vi "Dashboard Main.vi"() -> ()   [LabVIEW 2012]
uses:
  <vilib>/event_ctls.llb/eventvkey.ctl
  <vilib>/Utility/config.llb/Read Key (String).vi
  <vilib>/Utility/config.llb/Read Key (I32).vi
  <vilib>/Utility/config.llb/Write Key (String).vi
  <vilib>/Utility/config.llb/Write Key (I32).vi
  <vilib>/Utility/config.llb/NI_LVConfig.lvlib
panel:
  out "Mode":T1(ring)=enum."Auto Disabled"
  in  "Viewer":enum32{"Camera Image", "Variables"}(tab)
  out "Mbps":dbl format="%#.1g"
  in  "Enable":bool=TRUE
  in  "DB Camera Config":bool
  out "Mbps":bool
  out "fps":dbl format="%#.1g"
  out "Image Error Message":string="Timeout in Camera Communications"
  out "Camera Image":T2(plugin-control)
  out "Camera Image 2":T2(plugin-control)
  in  "Camera Settings":T3={"Frame Rate"=15, "Compression"=30, "Size"=1} {"Frame Rate" scale=1.0..30.0; "Size" items=["640x480", "320x240", "160x120"]}
  out "Camera IP 2":string
  out "Camera IP":string
  out "fps 2":dbl format="%#.1g"
  out "Mbps 2":dbl format="%#.1g"
  in  "Enable 2":bool=TRUE
  in  "FR":i32=15
  out "Tree":string(tree)
  in  "Dashboard Tab":enum32{"Operation", "Test", "Checklist"}(tab)
  in  "Auton Selector":T4(radio)
  in  "Auton Refresh":bool
  out "AutonFiles":string[](array[string])
  out "Refnum out":T2(plugin-control)
  in  "Score Limits":T5={"Rect Coverage"=60.0, "X Edge Strength"=40.0, "Y Edge Strength"=60.0, "Center"=75.0, "Outer"=75.0}
  in  "Range":cluster{"Lower value":sgl, "Upper value":sgl}={"Lower value"=150.0, "Upper value"=255.0}
  out "Out Circle Info":cluster{dbl, dbl}
  out "Out Target Info":cluster{"X":dbl, "Y":dbl, "Distance (ft)":dbl}
  in  "Slider":dbl(slide) scale=0.0..100.0 scale format="%#_3g"
  in  "On/Off":bool caption="Solenoid"
  in  "Test Name":u16(ring) items=["Select the test to run...", "Example Test", "-------------------------------", "List of tests is built in robot code.", "Replace with your own automated tests."]
  in  "Test Tree":string(tree)
  in  "Motor":cluster{"Value":dbl, "Enable":bool} {"Value" scale=-1.0..1.0 scale format="%#_3g"}
  out "Progress":T6 {"Test Progress" scale=0.0..100.0}
  in  "Rev/Fwd":cluster{"Forward":bool, "Reverse":bool}
  in  "Ring":u16(ring) items=["Auto", "Fixed indoor", "Fixed outdoor 1", "Fixed outdoor 2", "Fixed fluorescent 1", "Fixed fluorescent 2", "Hold current"]
  in  "Listbox":i32(listbox)
  out "Robot IP":string
  out "Battery Value":dbl(slide) scale=0.0..14.0 scale format="%#_2e"
  out "Battery":sgl(graph)
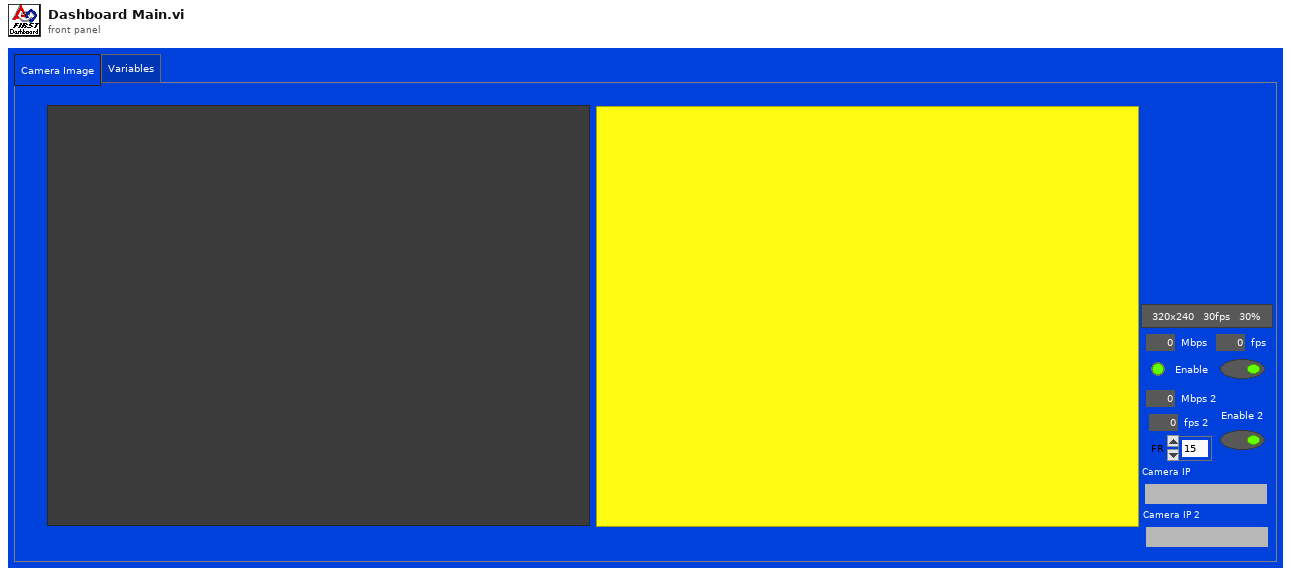
[diagram p1: front panel]
types:
  T1 = enum8{"Tele-Op Disabled", "Tele-Op Enabled", "Auto Disabled", "Auto Enabled", "Test Disabled", "Test Enabled", ""}
  T2 = typedef "IMAQ Image.ctl" = refnum<image>
  T3 = cluster{"Frame Rate":i32, "Compression":i32, "Size":u16}
  T4 = enum32{"Boolean 1", "Boolean 2", "Boolean 3", "Boolean 4", "Boolean 5", "Boolean 6", "Boolean 7", "Boolean 8", "Boolean 9", "Boolean 10"}
  T5 = cluster{"Rect Coverage":dbl, "X Edge Strength":dbl, "Y Edge Strength":dbl, "Center":dbl, "Outer":dbl}
  T6 = cluster{"Test Progress":u8, "Test Progress Text":string}
  T7 = typedef "Image Type" = u32
  T8 = cluster{"Competition mode":bool, "Robot Link":bool, "Autonomous":bool, "Enabled":bool, "E-Stop":bool, "Simulated":bool, "TestMode":bool, "Docked Window":bool}
  T9 = typedef "LVRectTypeDef.ctl" = cluster{"Left":i16, "Top":i16, "Right":i16, "Bottom":i16}
  T10 = typedef "NI_LVConfig.lvlib/Config Data RefNum.ctl" = refnum<k1>
  T11 = typedef "eventvkey.ctl" = enum16{"ASCII", "Enter", "Return", "Shift", "Ctrl", "Alt", "Cmd", "Opt", "Caps", "NumLock", "Clear", "Break", "Up", "Down", "Left", "Right", "Insert", "Delete", "Home", "End", "PageUp", "PageDown", "Escape", "Help", "Pause", "ScrollLock", "F1", "F2", "F3", "F4", "F5", "F6", "F7", "F8", "F9", "F10", "F11", "F12", "F13", "F14", "F15", "F16", "F17", "F18", "F19", "F20", "F21", "F22", "F23", "F24", "Play", "VolumeUp", "VolumeDown", "Mute", "Two Byte Char"}
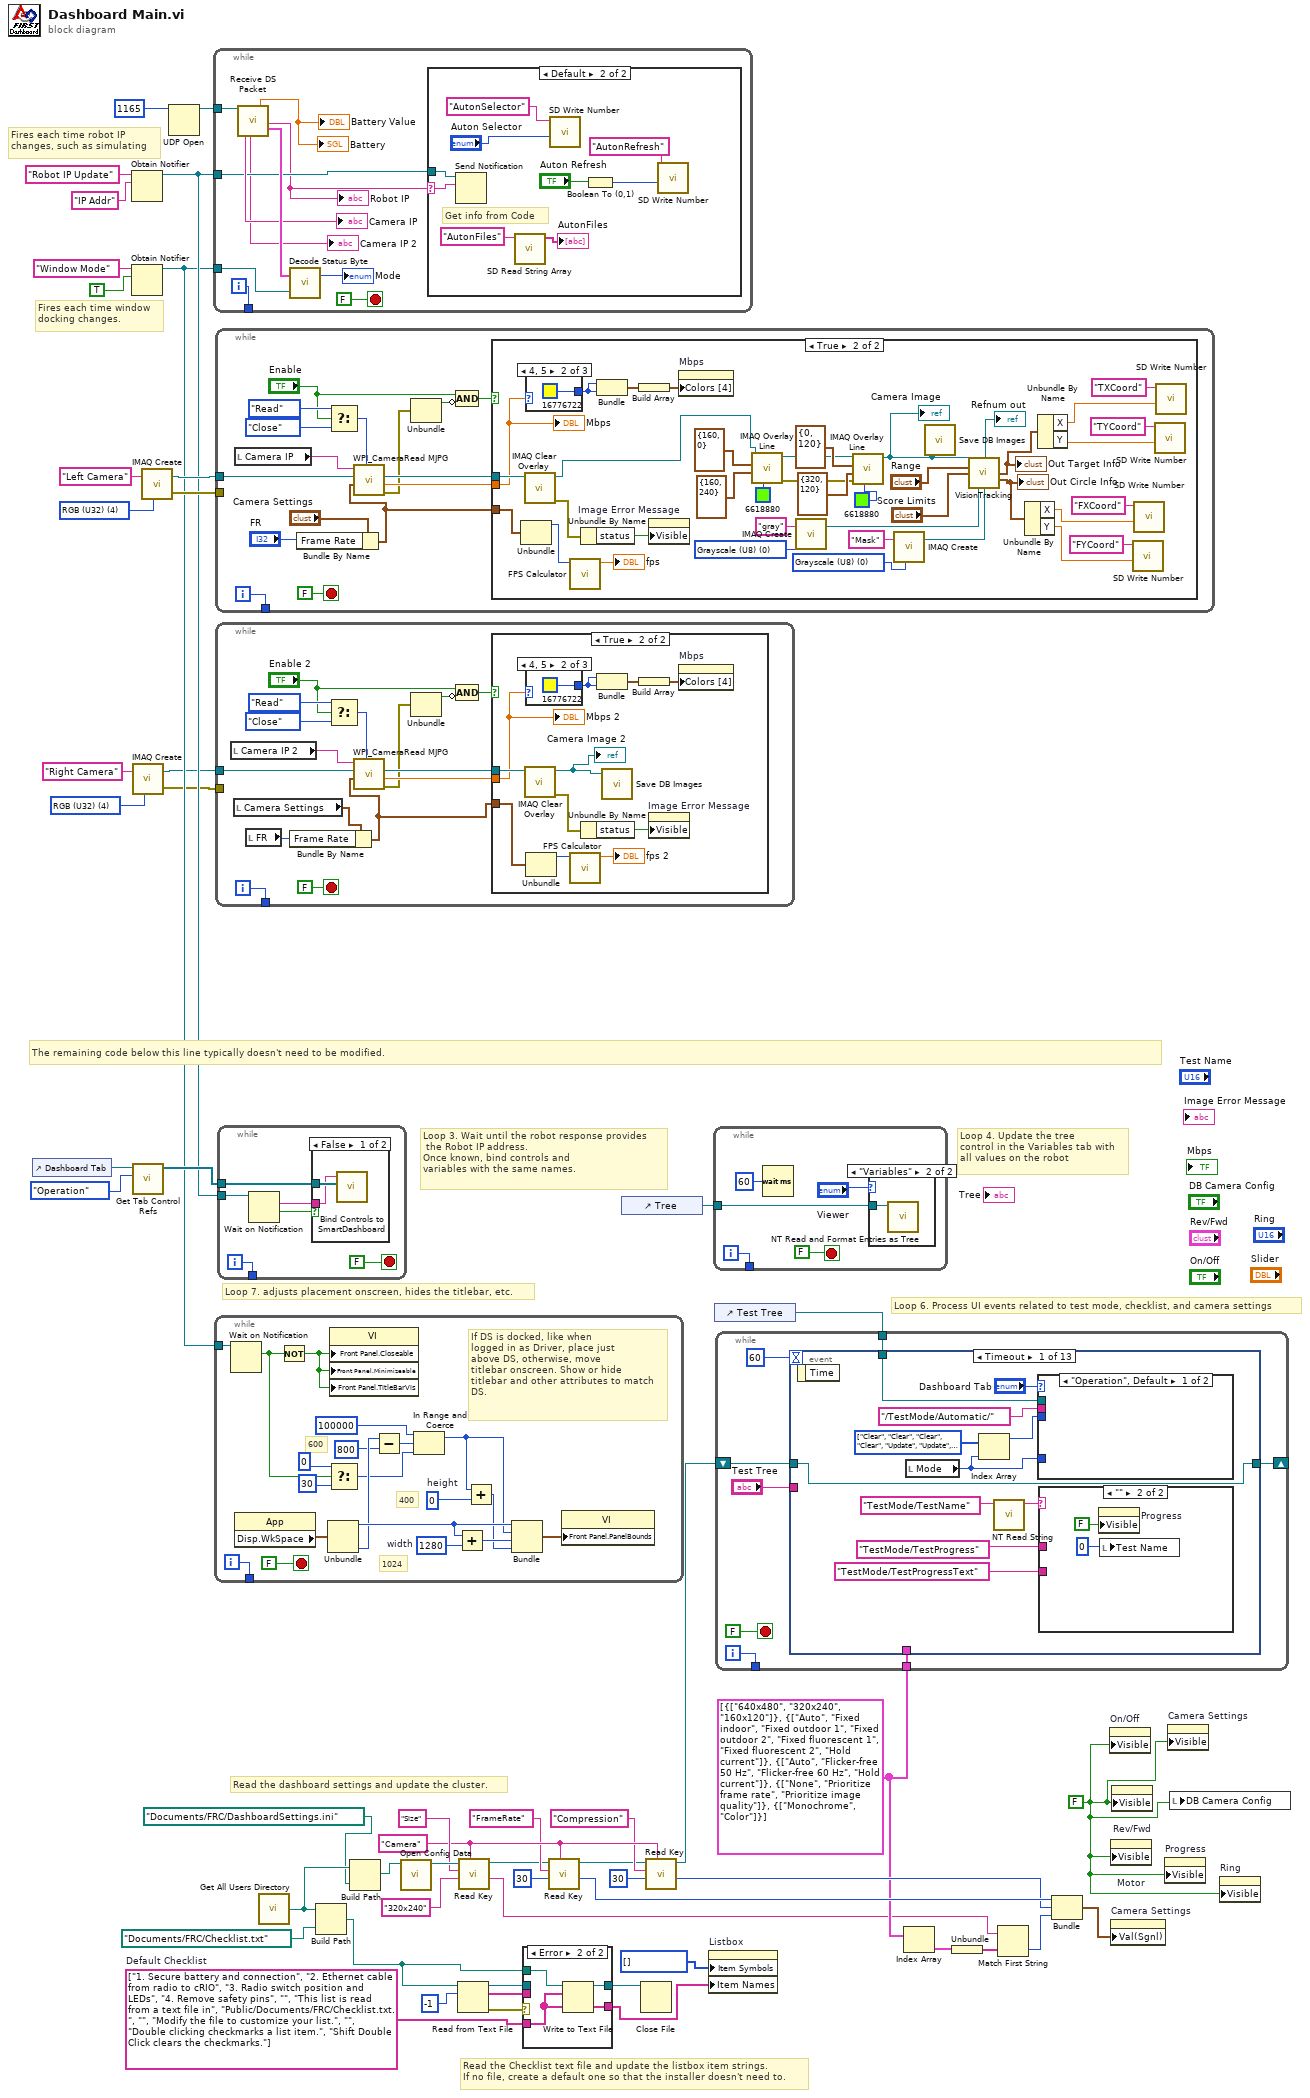
[diagram p0: block diagram]
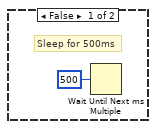
[diagram p2: hidden frame]
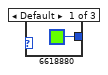
[diagram p3: hidden frame]
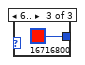
[diagram p4: hidden frame]
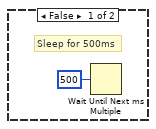
[diagram p6: hidden frame]
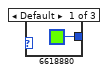
[diagram p7: hidden frame]
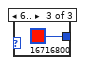
[diagram p8: hidden frame]
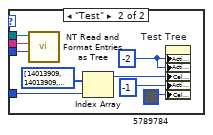
[diagram p10: hidden frame]
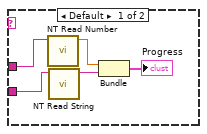
[diagram p11: hidden frame]
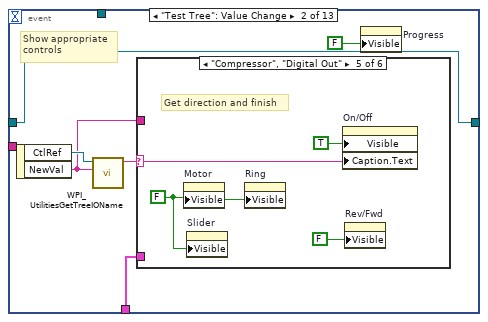
[diagram p12: hidden frame]
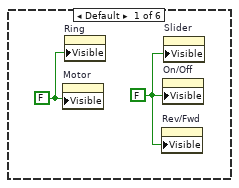
[diagram p13: hidden frame]
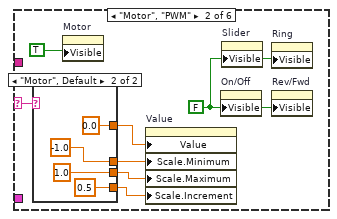
[diagram p14: hidden frame]
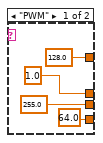
[diagram p15: hidden frame]
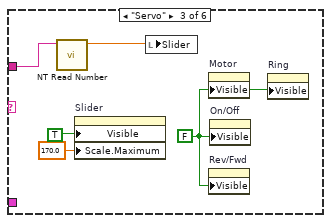
[diagram p16: hidden frame]
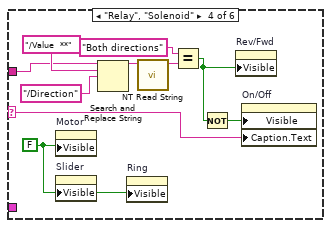
[diagram p17: hidden frame]
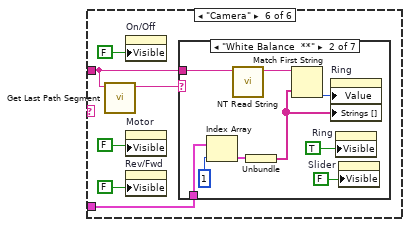
[diagram p18: hidden frame]
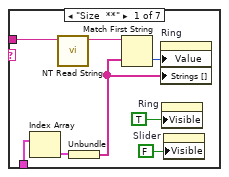
[diagram p19: hidden frame]
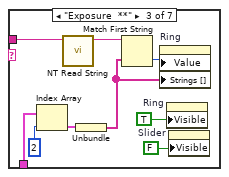
[diagram p20: hidden frame]
diagram:
  w3 = T7 4 items=["Grayscale (U8)", "Grayscale (I16)", "Grayscale (SGL)", "Complex (CSG)", "RGB (U32)", "HSL (U32)", "RGB (U64)"] ("Image Type")
  w25 = "Camera"
  w17 = cluster{string[]}[] [{["640x480", "320x240", "160x120"]}, {["Auto", "Fixed indoor", "Fixed outdoor 1", "Fixed outdoor 2", "Fixed fluorescent 1", "Fixed fluorescent 2", "Hold current"]}, {["Auto", "Flicker-free 50 Hz", "Flicker-free 60 Hz", "Hold current"]}, {["None", "Prioritize frame rate", "Prioritize image quality"]}, {["Monochrome", "Color"]}]
  w33 = string[] ["1. Secure battery and connection", "2. Ethernet cable from radio to cRIO", "3. Radio switch position and LEDs", "4. Remove safety pins", "", "This list is read from a text file in", "Public/Documents/FRC/Checklist.txt.", "", "Modify the file to customize your list.", "", "Double clicking checkmarks a list item.", "Shift Double Click clears the checkmarks."]  # Default Checklist
  w31 = FALSE ("Visible")
  w52 = T7 4 items=["Grayscale (U8)", "Grayscale (I16)", "Grayscale (SGL)", "Complex (CSG)", "RGB (U32)", "HSL (U32)", "RGB (U64)"] ("Image Type")
  # "Fires each time robot IP\nchanges, such as simulating"
  # "Fires each time window\ndocking changes."
  # "Read the Checklist text file and update the listbox item strings.\nIf no file, create a default one so that the installer doesn't need to."
  # "The remaining code below this line typically doesn't need to be modified."
  # "Loop 6. Process UI events related to test mode, checklist, and camera settings"
  # "Read the dashboard settings and update the cluster."
  # "Loop 4. Update the tree\ncontrol in the Variables tab with\nall values on the robot"
  # "Loop 3. Wait until the robot response provides\n the Robot IP address.\nOnce known, bind controls and\nvariables with the same names."
  # "Loop 7. adjusts placement onscreen, hides the titlebar, etc."
  n1 = control-ref of="Dashboard Tab"() -> (w47:refnum<vi>)
  n2 = Obtain Notifier(name (unnamed)="Robot IP Update", notification data type="IP Addr" ("name (unnamed)")) -> (notifier out=w44:refnum<notifier>)  [unwired: 2 in, 2 out]
  n3 = Obtain Notifier(name (unnamed)="Window Mode", notification data type=TRUE) -> (notifier out=w37:refnum<notifier>)  [unwired: 2 in, 2 out]
  n4 = call "IMAQ Create"("Image Name"="Right Camera", "Image Type"=w3) -> ("New Image"=w2:T2, "error out"=w1:errorcluster)  [unwired: 2 in, 1 out]
  n5 = call <vilib>:"Get Tab Control Refs.vi"("Page Index"=enum32{"Operation", "Test"}."Operation" ("Dashboard Tab"), "TabControl in"=w47) -> ("ControlsOnPage"=w48:refnum<vi>[])  [unwired: 9 in]
  n6 = call "IMAQ Create"("Image Name"="Left Camera", "Image Type"=w52) -> ("New Image"=w50:T2, "error out"=w49:errorcluster)  [unwired: 2 in, 1 out]
  n7 = UDP Open(11:u16 1165 ("port")) -> (port=w53:refnum<k16>)  [unwired: 2 in, 4 out]
  n8 = while {
    tunnel: w53 -> [w63]
    tunnel: w44 -> [w57]
    tunnel: w37 -> [w61]
    tunnel: [w58] -> _
    i -> [w58]
    stop <- FALSE stop-if-true
    n9 = call "Receive DS Packet.vi"("Recv Socket"=w63) -> ("Camera IP Address"=→"Camera IP":string, "Camera IP Address 2"=→"Camera IP 2":string, "Battery"=→"Battery" →"Battery Value":sgl, "Robot IP Address"=w56:string, "Status"=w64:T8)  [unwired: 8 in, 6 out]
    "Robot IP" <- w56
    n10 = call "Decode Status Byte.vi"("Window Mode Notifier"=w61, "Status"=w64) -> ("Mode"=→"Mode":T1)  [unwired: 1 out]
    n11 = case shown="Default" w56 {
      selector: w56 -> [_ w73]
      tunnel: w57 -> [_ w74]
      frame "0.0.0.0" {
        # "Robot not responding, don't poll the variables"
      }
      frame Default {
        # "Get info from Code"
        n12 = Send Notification(notification=w73, notifier=w74) -> ()  [unwired: 1 in, 2 out]
        n13 = call <vilib>:"SD Read String Array.vi"("Name"="AutonFiles") -> ("String Array"=→"AutonFiles":string[])  [unwired: 9 in, 1 out]
        n14 = call <vilib>:"SD Write Number.vi"("Numeric"="Auton Selector", "Name"="AutonSelector") -> ()  [unwired: 8 in, 2 out]
        n15 = Boolean To (0,1)(Boolean="Auton Refresh") -> (0, 1=w67:i16)
        n16 = call <vilib>:"SD Write Number.vi"("Numeric"=w67, "Name"="AutonRefresh") -> ()  [unwired: 8 in, 2 out]
      }
    }
  }
  n17 = while {
    tunnel: w37 -> [w93]
    tunnel: [w91] -> _
    i -> [w91]
    stop <- FALSE stop-if-true
    w83 = 1280  # width
    w86 = 0  # height
    # "600"
    # "1024"
    # "400"
    # "If DS is docked, like when\nlogged in as Driver, place just\nabove DS, otherwise, move\ntitlebar onscreen. Show or hide\ntitlebar and other attributes to match\nDS."
    n18 = Wait on Notification(notifier=w93) -> (notification=w78:bool)  [unwired: 3 in, 3 out]
    n19 = property class="App"() -> ("Disp.WkSpace"=w89:T9)  [unwired: 2 in, 2 out]
    n20 = Not(x=w78) -> (.not. x?=w92:bool)
    n21 = Unbundle(w89) -> ("Left"=w87:i16, "Bottom"=w84:i16)  [unwired: 2 out]
    n22 = Select(t=0, s=w78, f=30) -> (s? t:f=w77:i32)
    n23 = property class="VI"("Front Panel.Closeable"=w92, "Front Panel.Minimizeable"=w92, "Front Panel.TitleBarVis"=w92) -> ()  [unwired: 2 in, 2 out]
    n24 = Subtract(x=w84, y=800) -> (x-y=w81:i32)
    n25 = In Range and Coerce(upper limit=100000, x=w81, lower limit=w77) -> (coerced(x)=w75:i32)  [unwired: 1 out]
    n26 = Add(x=w87, y=w83) -> (x+y=w88:i32)
    n27 = Add(x=w75, y=w86) -> (x+y=w85:i32)
    n28 = Bundle("Left"=w87, w75, w88, w85) -> (w90:cluster{"Left":i16, i32, i32, i32})  [unwired: 1 out]
    n29 = property class="VI"("Front Panel.PanelBounds"=w90) -> ()  [unwired: 2 in, 2 out]
  }
  n30 = while {
    tunnel: w50 -> [w107]
    tunnel: w49 -> [_]
    tunnel: [w109] -> _
    i -> [w109]
    stop <- FALSE stop-if-true
    n31 = local read "Camera IP"() -> (w108:string)
    n32 = Bundle By Name(cluster="Camera Settings", "Frame Rate"="FR") -> (w95:T3)
    n33 = Select(t=enum16{"Read", "Reopen", "Close"}."Read" ("Operation"), s="Enable", f=enum16{"Read", "Reopen", "Close"}."Close" ("Operation")) -> (s? t:f=w102:enum16{"Read", "Reopen", "Close"})
    n34 = call <vilib>:"WPI_CameraRead MJPG.vi"("Operation"=w102, "Camera Settings"=w95, "Image"=w107, "address"=w108) -> ("error out"=w101:errorcluster, "Bandwidth (kbps)"=w105:dbl, "Image Out"=w106:T2)  [unwired: 5 in]
    n35 = Unbundle(w101) -> ("status"=w99:bool)  [unwired: 2 out]
    n36 = Compound Arithmetic op=AND("Enable", invert w99) -> (w98:bool)
    n37 = case shown="True" w98 {
      tunnel: w95 -> [_ w142]
      tunnel: w106 -> [_ w145]
      tunnel: w105 -> [_ w144]
      frame False {
        # "Sleep for 500ms"
        n38 = Wait Until Next ms Multiple(millisecond multiple=u32 500) -> ()  [unwired: 1 out]
      }
      frame True {
        w126 = T7 0 items=["Grayscale (U8)", "Grayscale (I16)", "Grayscale (SGL)", "Complex (CSG)", "RGB (U32)", "HSL (U32)", "RGB (U64)", "Grayscale (U16)"] ("Image Type")
        w128 = T7 0 items=["Grayscale (U8)", "Grayscale (I16)", "Grayscale (SGL)", "Complex (CSG)", "RGB (U32)", "HSL (U32)", "RGB (U64)", "Grayscale (U16)"] ("Image Type")
        n39 = Unbundle(w142) -> ("Frame Rate"=w133:i32)  [unwired: 2 out]
        n40 = call "IMAQ Clear Overlay"("Image"=w145) -> ("error out"=w149:errorcluster, "Image Out"=w134:T2)  [unwired: 2 in, 7 out]
        n41 = case shown="4, 5" w144 {
          tunnel: [u32 6618880 ("Color Box") u32 16776722 ("Color Box") u32 16716800 ("Color Box")] -> w146
          frame Default {
          }
          frame 4, 5 {
          }
          frame 6.. {
          }
        }
        n42 = call "FPS Calculator.vi"("Average Count"=w133) -> ("fps"=→"fps":dbl)  [unwired: 10 in]
        n43 = Unbundle By Name(w149) -> ("status"=w150:bool)
        n44 = Bundle("Color Box"=w146, "Color Box"=w146) -> (w148:cluster{"Color Box":u32, "Color Box":u32})  [unwired: 1 out]
        n45 = Build Array(w148) -> (w147:cluster{"Color Box":u32, "Color Box":u32}[])
        n46 = property on="Image Error Message" class="Str"("Visible"=w150) -> ()  [unwired: 2 in, 2 out]
        n47 = property on="Mbps" class="Bool (strict)"("Colors [4]"=w147) -> ()  [unwired: 2 in, 2 out]
        n48 = call "IMAQ Overlay Line"("Color"=u32 6618880, "End Point"=cluster{"X":i32, "Y":i32} {"X"=160, "Y"=240}, "Start Point"=cluster{"X":i32, "Y":i32} {"X"=160, "Y"=0}, "Image"=w134) -> ("error out"=w139:errorcluster, "Image Out"=w138:T2)  [unwired: 6 in]
        n49 = call "IMAQ Create"("Image Name"="gray", "Image Type"=w128) -> ("New Image"=w124:T2)  [unwired: 3 in, 1 out]
        n50 = call "IMAQ Overlay Line"("Color"=u32 6618880, "error in (no error)"=w139, "End Point"=cluster{"X":i32, "Y":i32} {"X"=320, "Y"=120}, "Start Point"=cluster{"X":i32, "Y":i32} {"X"=0, "Y"=120}, "Image"=w138) -> ("Image Out"=w131:T2)  [unwired: 5 in, 1 out]
        "Camera Image" <- w131
        n51 = call "IMAQ Create"("Image Name"="Mask", "Image Type"=w126) -> ("New Image"=w125:T2)  [unwired: 3 in, 1 out]
        n52 = call "Save DB Images.vi"("Image"=w131) -> ()  [unwired: 2 in, 1 out]
        n53 = call "VisionTracking.vi"("Refnum in"=w131, "Range"="Range", "Score Limits"="Score Limits", "New Image 2"=w124, "New Image"=w125) -> ("Refnum out"=→"Refnum out":T2, "Out Target Info"=w121:cluster{"X":dbl, "Y":dbl, "Distance (ft)":dbl}, "Out Cirlcle Info"=w114:cluster{"X":dbl, "Y":dbl})  [unwired: 8 in]
        "Out Target Info" <- w121
        "Out Circle Info" <- w114
        n54 = Unbundle By Name(w114) -> ("X"=w113:dbl, "Y"=w112:dbl)
        n55 = Unbundle By Name(w121) -> ("X"=w118:dbl, "Y"=w117:dbl)
        n56 = call <vilib>:"SD Write Number.vi"("Numeric"=w112, "Name"="FYCoord") -> ()  [unwired: 8 in, 2 out]
        n57 = call <vilib>:"SD Write Number.vi"("Numeric"=w113, "Name"="FXCoord") -> ()  [unwired: 8 in, 2 out]
        n58 = call <vilib>:"SD Write Number.vi"("Numeric"=w117, "Name"="TYCoord") -> ()  [unwired: 8 in, 2 out]
        n59 = call <vilib>:"SD Write Number.vi"("Numeric"=w118, "Name"="TXCoord") -> ()  [unwired: 8 in, 2 out]
        "Mbps" <- w144
      }
    }
  }
  n60 = while {
    tunnel: w2 -> [w166]
    tunnel: [w168] -> _
    tunnel: w1 -> [_]
    i -> [w168]
    stop <- FALSE stop-if-true
    n61 = local read "Camera IP 2"() -> (w167:string)
    n62 = local read "Camera Settings"() -> (w155:T3)
    n63 = local read "FR"() -> (w156:i32)
    n64 = Bundle By Name(cluster=w155, "Frame Rate"=w156) -> (w154:T3)
    n65 = Select(t=enum16{"Read", "Reopen", "Close"}."Read" ("Operation"), s="Enable 2", f=enum16{"Read", "Reopen", "Close"}."Close" ("Operation")) -> (s? t:f=w161:enum16{"Read", "Reopen", "Close"})
    n66 = call <vilib>:"WPI_CameraRead MJPG.vi"("Operation"=w161, "Camera Settings"=w154, "Image"=w166, "address"=w167) -> ("error out"=w160:errorcluster, "Bandwidth (kbps)"=w164:dbl, "Image Out"=w165:T2)  [unwired: 5 in]
    n67 = Unbundle(w160) -> ("status"=w158:bool)  [unwired: 2 out]
    n68 = Compound Arithmetic op=AND("Enable 2", invert w158) -> (w157:bool)
    n69 = case shown="True" w157 {
      tunnel: w154 -> [_ w173]
      tunnel: w165 -> [_ w176]
      tunnel: w164 -> [_ w175]
      frame False {
        # "Sleep for 500ms"
        n70 = Wait Until Next ms Multiple(millisecond multiple=u32 500) -> ()  [unwired: 1 out]
      }
      frame True {
        n71 = call "IMAQ Clear Overlay"("Image"=w176) -> ("error out"=w180:errorcluster, "Image Out"=w171:T2)  [unwired: 2 in, 7 out]
        "Camera Image 2" <- w171
        n72 = case shown="4, 5" w175 {
          tunnel: [u32 6618880 ("Color Box") u32 16776722 ("Color Box") u32 16716800 ("Color Box")] -> w177
          frame Default {
          }
          frame 4, 5 {
          }
          frame 6.. {
          }
        }
        n73 = Unbundle(w173) -> ("Frame Rate"=w172:i32)  [unwired: 2 out]
        n74 = call "FPS Calculator.vi"("Average Count"=w172) -> ("fps"=→"fps 2":dbl)  [unwired: 10 in]
        n75 = Unbundle By Name(w180) -> ("status"=w181:bool)
        n76 = Bundle("Color Box"=w177, "Color Box"=w177) -> (w179:cluster{"Color Box":u32, "Color Box":u32})  [unwired: 1 out]
        n77 = call "Save DB Images.vi"("Image"=w171) -> ()  [unwired: 2 in, 1 out]
        n78 = Build Array(w179) -> (w178:cluster{"Color Box":u32, "Color Box":u32}[])
        n79 = property on="Image Error Message" class="Str"("Visible"=w181) -> ()  [unwired: 2 in, 2 out]
        n80 = property on="Mbps" class="Bool (strict)"("Colors [4]"=w178) -> ()  [unwired: 2 in, 2 out]
        "Mbps 2" <- w175
      }
    }
  }
  n81 = while {
    tunnel: w48 -> [w190]
    tunnel: w44 -> [w187]
    tunnel: [w185] -> _
    i -> [w185]
    stop <- FALSE stop-if-true
    n82 = Wait on Notification(notifier=w187) -> (notification=w186:string, timed out?=w188:bool)  [unwired: 3 in, 2 out]
    n83 = case shown="False" w188 {
      tunnel: w190 -> [w192 _]
      tunnel: w186 -> [w191 _]
      frame False {
        n84 = call <vilib>:"Bind Controls to SmartDashboard.vi"("Bound Control Refs"=w192, "Server IP Address"=w191) -> ()  [unwired: 10 in]
      }
      frame True {
      }
    }
  }
  n85 = call "Get All Users Directory.vi"() -> ("All User Path"=w30:path)
  n86 = Build Path(base path=w30, name or relative path=path "Documents/FRC/Checklist.txt") -> (appended path=w34:path)
  n87 = Build Path(base path=w30, name or relative path=path "Documents/FRC/DashboardSettings.ini") -> (appended path=w29:path)
  n88 = call <vilib>:"Open Config Data.vi"("configuration file path"=w29) -> ("refnum"=w28:T10)  [unwired: 8 in, 2 out]
  n89 = Read from Text File(file (use dialog)=w34, count=-1 ("timeout ms (25000)")) -> (refnum out=w12:refnum<file>, text=w35:string[], error out=w36:errorcluster)  [unwired: 2 in, 1 out]
  n90 = call-poly <vilib>:"Read Key.vi"("section"=w25, "default value"="320x240", "key"="Size", "refnum"=w28) -> ("value"=w15:string, "refnum out"=w10:T10)  [unwired: 2 in, 4 out]
  n91 = case shown="Error" w36 {
    tunnel: w35 -> [w194 _]
    tunnel: [w194 w196] -> w32
    tunnel: w33 -> [_ w196]
    tunnel: w34 -> [_ w197]
    tunnel: [w193 w195] -> w11
    tunnel: w12 -> [w193 _]
    frame No Error {
    }
    frame Error {
      n92 = Write to Text File(file (use dialog)=w197, text=w196) -> (refnum out=w195:refnum<file>)  [unwired: 2 in, 2 out]
    }
  }
  n93 = call-poly <vilib>:"Read Key.vi"("section"=w25, "default value"=30, "key"="FrameRate", "refnum"=w10) -> ("value"=w20:i32, "refnum out"=w9:T10)  [unwired: 1 in, 5 out]
  n94 = control-ref of="Tree"() -> (w6:refnum<vi>)
  n95 = Close File(refnum=w11) -> ()  [unwired: 1 in, 2 out]
  n96 = call-poly <vilib>:"Read Key.vi"("section"=w25, "default value"=30, "key"="Compression", "refnum"=w9) -> ("value"=w19:i32, "refnum out"=w7:T10)  [unwired: 1 in, 5 out]
  n97 = property on="Listbox" class="LstBox (strict)"("Item Symbols"=i32[] [], "Item Names"=w32) -> ()  [unwired: 2 in, 2 out]
  n98 = while {
    tunnel: [w199] -> _
    tunnel: w6 -> [w198]
    i -> [w199]
    stop <- FALSE stop-if-true
    n99 = Wait (ms)(milliseconds to wait=u32 60) -> ()  [unwired: 1 out]
    n100 = case shown="\"Variables\"" "Viewer" {
      tunnel: w198 -> [_ w203]
      frame Default {
      }
      frame "Variables" {
        n101 = call <vilib>:"NT Read and Format Entries as Tree.vi"("Tree Refnum"=w203) -> ()  [unwired: 9 in, 2 out]
      }
    }
  }
  n102 = control-ref of="Test Tree"() -> (w5:refnum<vi>)
  n103 = while {
    tunnel: w17 -> [w208]
    shift-right: [w207] -> _
    shift-left: w7 -> [w206]
    tunnel: [w205] -> _
    tunnel: w5 -> [w204]
    i -> [w205]
    stop <- FALSE stop-if-true
    n104 = event shown="[0] Timeout" {
      selector: _ -> [_ _ _ _ _ _ _ _ _ _ _ _ _]
      dyn-events: _ -> [_ _ _ _ _ _ _ _ _ _ _ _ _]
      timeout: u32 60 ("milliseconds to wait") -> [_ _ _ _ _ _ _ _ _ _ _ _ _]
      tunnel: w204 -> [w218 _ _ _ _ _ _ _ _ _ _ _ _]
      tunnel: "Test Tree" -> [_ _ _ _ _ _ _ _ w412 w420 w422 w426 w434]
      tunnel: w208 -> [_ w240 _ _ _ _ w376 w406 _ _ _ _ _]
      tunnel: [w212 w239 _ w342 w350 w362 w375 w399 w411 w418 w421 w425 w433] -> w207
      tunnel: w206 -> [w212 w239 _ w342 w350 w362 w374 w399 w411 w418 w421 w425 w433]
      event Timeout {
        w217 = enum16{"Update", "Clear"}[] [enum."Clear", enum."Clear", enum."Clear", enum."Clear", enum."Update", enum."Update", enum."Clear"] items=["Update", "Clear"]
        n105 = event-data() -> ()  [unwired: 1 in, 1 out]
        n106 = local read "Mode"() -> (w215:T1)
        n107 = Index Array(array=w217, index=w215) -> (element=w216:enum16{"Update", "Clear"})
        n108 = call <vilib>:"NT Read String.vi"("Name"="TestMode/TestName") -> ("String"=w221:string)  [unwired: 9 in, 1 out]
        n109 = case shown="\"Operation\", Default" "Dashboard Tab" {
          tunnel: w218 -> [_ w231]
          tunnel: "/TestMode/Automatic/" ("Name Pattern") -> [_ w230]
          tunnel: w216 -> [_ w229]
          tunnel: w215 -> [_ w227]
          frame "Operation", Default {
          }
          frame "Test" {
            w226 = -2 ("Active Item:Row Number")
            n110 = call <vilib>:"NT Read and Format Entries as Tree.vi"("Operation"=w229, "Name Pattern"=w230, "Tree Refnum"=w231) -> ()  [unwired: 7 in, 2 out]
            n111 = Index Array(array=u32[] [14013909, 14013909, 14013909, 14013909, 14013909, 16777215, 14013909], index=w227) -> (element=w225:u32)
            n112 = property on="Test Tree" class="Tree (strict)"("Active Item Row Number"=w226, "ActiveColNum"=w226, "CellBG"=w225, "Active Item Row Number"=-1 ("Active Item:Row Number"), "CellBG"=u32 5789784 ("Color Box")) -> ()  [unwired: 2 in, 2 out]
          }
        }
        n113 = case shown="\"\"" w221 {
          tunnel: "TestMode/TestProgress" ("Name") -> [w233 _]
          tunnel: "TestMode/TestProgressText" ("Name") -> [w232 _]
          frame Default {
            n114 = call <vilib>:"NT Read Number.vi"("Name"=w233) -> ("Numeric"=w234:dbl)  [unwired: 9 in, 1 out]
            n115 = call <vilib>:"NT Read String.vi"("Name"=w232) -> ("String"=w235:string)  [unwired: 9 in, 1 out]
            n116 = Bundle("Numeric"=w234, "String"=w235) -> (→"Progress":cluster{"Numeric":dbl, "String":string})  [unwired: 1 in]
          }
          frame "" {
            n117 = property on="Progress" class="Clust (strict)"("Visible"=FALSE) -> ()  [unwired: 2 in, 2 out]
            n118 = local write "Test Name"(u16 0) -> ()
          }
        }
      }
      event "Test Tree": Value Change {
        # "Show appropriate\ncontrols"
        n119 = event-data() -> ("CtlRef"=w243:refnum<vi>, "NewVal"=w241:string)  [unwired: 1 in]
        n120 = call <vilib>:"WPI_UtilitiesGetTreeIOName.vi"("NewVal"=w241, "TreeControl in"=w243) -> ("I/O Name"=w244:string)  [unwired: 9 in]
        n121 = case shown="\"Compressor\", \"Digital Out\"" w244 {
          selector: w244 -> [_ w251 _ w269 w278 _]
          tunnel: w241 -> [_ _ w266 w268 _ w285]
          tunnel: w240 -> [_ _ _ _ _ w284]
          frame Default {
            w246 = FALSE ("Visible")
            w245 = FALSE ("Visible")
            n122 = property on="Motor" class="Clust (strict)"("Visible"=w245) -> ()  [unwired: 2 in, 2 out]
            n123 = property on="Ring" class="Ring (strict)"("Visible"=w245) -> ()  [unwired: 2 in, 2 out]
            n124 = property on="Rev/Fwd" class="Clust (strict)"("Visible"=w246) -> ()  [unwired: 2 in, 2 out]
            n125 = property on="On/Off" class="Bool (strict)"("Visible"=w246) -> ()  [unwired: 2 in, 2 out]
            n126 = property on="Slider" class="Slide (strict)"("Visible"=w246) -> ()  [unwired: 2 in, 2 out]
          }
          frame "Motor", "PWM" {
            w252 = FALSE ("Visible")
            n127 = case shown="\"Motor\", Default" w251 {
              tunnel: [1.0 ("Value") -1.0 ("Value")] -> w250
              tunnel: [255.0 ("Value") 1.0 ("Value")] -> w249
              tunnel: [128.0 ("Value") 0.0 ("Value")] -> w248
              tunnel: [64.0 ("Value") 0.5 ("Value")] -> w247
              frame "PWM" {
              }
              frame "Motor", Default {
              }
            }
            n128 = property on="Motor" class="Clust (strict)"("Visible"=TRUE) -> ()  [unwired: 2 in, 2 out]
            n129 = property on="Value" class="Slide (strict)"("Value"=w248, "Scale.Minimum"=w250, "Scale.Maximum"=w249, "Scale.Increment"=w247) -> ()  [unwired: 2 in, 2 out]
            n130 = property on="On/Off" class="Bool (strict)"("Visible"=w252) -> ()  [unwired: 2 in, 2 out]
            n131 = property on="Slider" class="Slide (strict)"("Visible"=w252) -> ()  [unwired: 2 in, 2 out]
            n132 = property on="Ring" class="Ring (strict)"("Visible"=w252) -> ()  [unwired: 2 in, 2 out]
            n133 = property on="Rev/Fwd" class="Clust (strict)"("Visible"=w252) -> ()  [unwired: 2 in, 2 out]
          }
          frame "Servo" {
            w264 = FALSE ("Visible")
            n134 = call <vilib>:"NT Read Number.vi"("Name"=w266) -> ("Numeric"=w265:dbl)  [unwired: 9 in, 1 out]
            n135 = property on="Slider" class="Slide (strict)"("Visible"=TRUE, "Scale.Maximum"=170.0 ("Scale.Range:Maximum")) -> ()  [unwired: 2 in, 2 out]
            n136 = local write "Slider"(w265) -> ()
            n137 = property on="Motor" class="Clust (strict)"("Visible"=w264) -> ()  [unwired: 2 in, 2 out]
            n138 = property on="Rev/Fwd" class="Clust (strict)"("Visible"=w264) -> ()  [unwired: 2 in, 2 out]
            n139 = property on="On/Off" class="Bool (strict)"("Visible"=w264) -> ()  [unwired: 2 in, 2 out]
            n140 = property on="Ring" class="Ring (strict)"("Visible"=w264) -> ()  [unwired: 2 in, 2 out]
          }
          frame "Relay", "Solenoid" {
            w267 = FALSE ("Visible")
            n141 = property on="Motor" class="Clust (strict)"("Visible"=w267) -> ()  [unwired: 2 in, 2 out]
            n142 = property on="Slider" class="Slide (strict)"("Visible"=w267) -> ()  [unwired: 2 in, 2 out]
            n143 = Search and Replace String(input string=w268, search string="/Value  **", replace string="/Direction") -> (result string=w274:string)  [unwired: 5 in, 3 out]
            n144 = property on="Ring" class="Ring (strict)"("Visible"=w267) -> ()  [unwired: 2 in, 2 out]
            n145 = call <vilib>:"NT Read String.vi"("Name"=w274) -> ("String"=w272:string)  [unwired: 9 in, 1 out]
            n146 = Equal?(x="Both directions", y=w272) -> (x = y?=w270:bool)
            n147 = Not(x=w270) -> (.not. x?=w271:bool)
            n148 = property on="Rev/Fwd" class="Clust (strict)"("Visible"=w270) -> ()  [unwired: 2 in, 2 out]
            n149 = property on="On/Off" class="Bool (strict)"("Visible"=w271, "Caption.Text"=w269) -> ()  [unwired: 2 in, 2 out]
          }
          frame "Compressor", "Digital Out" {
            w277 = FALSE ("Visible")
            # "Get direction and finish"
            n150 = property on="Motor" class="Clust (strict)"("Visible"=w277) -> ()  [unwired: 2 in, 2 out]
            n151 = property on="Slider" class="Slide (strict)"("Visible"=w277) -> ()  [unwired: 2 in, 2 out]
            n152 = property on="Ring" class="Ring (strict)"("Visible"=w277) -> ()  [unwired: 2 in, 2 out]
            n153 = property on="On/Off" class="Bool (strict)"("Visible"=TRUE, "Caption.Text"=w278) -> ()  [unwired: 2 in, 2 out]
            n154 = property on="Rev/Fwd" class="Clust (strict)"("Visible"=FALSE) -> ()  [unwired: 2 in, 2 out]
          }
          frame "Camera" {
            n155 = call <vilib>:"Get Last Path Segment.vi"("String in"=w285) -> ("String out"=w286:string)  [unwired: 10 in]
            n156 = property on="On/Off" class="Bool (strict)"("Visible"=FALSE) -> ()  [unwired: 2 in, 2 out]
            n157 = property on="Motor" class="Clust (strict)"("Visible"=FALSE) -> ()  [unwired: 2 in, 2 out]
            n158 = property on="Rev/Fwd" class="Clust (strict)"("Visible"=FALSE) -> ()  [unwired: 2 in, 2 out]
            n159 = case shown="\"White Balance  **\"" w286 {
              tunnel: w285 -> [w292 w301 w310 w319 w328 _ w334]
              tunnel: w284 -> [w290 w298 w307 w316 w325 _ _]
              frame "Size  **" {
                n160 = Index Array(array=w290) -> (element=w289:cluster{string[]})  [unwired: 1 in]
                n161 = call <vilib>:"NT Read String.vi"("Name"=w292) -> ("String"=w291:string)  [unwired: 9 in, 1 out]
                n162 = Unbundle(w289) -> (w287:string[])
                n163 = Match First String(2:w287, 3:w291) -> (0:w288:i32)  [unwired: 1 out]
                n164 = property on="Ring" class="Ring (strict)"("Value"=w288, "Strings []"=w287) -> ()  [unwired: 2 in, 2 out]
                n165 = property on="Ring" class="Ring (strict)"("Visible"=TRUE) -> ()  [unwired: 2 in, 2 out]
                n166 = property on="Slider" class="Slide (strict)"("Visible"=FALSE) -> ()  [unwired: 2 in, 2 out]
              }
              frame "White Balance  **" {
                n167 = Index Array(array=w298, index=1) -> (element=w299:cluster{string[]})
                n168 = call <vilib>:"NT Read String.vi"("Name"=w301) -> ("String"=w300:string)  [unwired: 9 in, 1 out]
                n169 = Unbundle(w299) -> (w296:string[])
                n170 = Match First String(2:w296, 3:w300) -> (0:w295:i32)  [unwired: 1 out]
                n171 = property on="Ring" class="Ring (strict)"("Value"=w295, "Strings []"=w296) -> ()  [unwired: 2 in, 2 out]
                n172 = property on="Ring" class="Ring (strict)"("Visible"=TRUE) -> ()  [unwired: 2 in, 2 out]
                n173 = property on="Slider" class="Slide (strict)"("Visible"=FALSE) -> ()  [unwired: 2 in, 2 out]
              }
              frame "Exposure  **" {
                n174 = Index Array(array=w307, index=2) -> (element=w308:cluster{string[]})
                n175 = call <vilib>:"NT Read String.vi"("Name"=w310) -> ("String"=w309:string)  [unwired: 9 in, 1 out]
                n176 = Unbundle(w308) -> (w304:string[])
                n177 = Match First String(2:w304, 3:w309) -> (0:w305:i32)  [unwired: 1 out]
                n178 = property on="Ring" class="Ring (strict)"("Value"=w305, "Strings []"=w304) -> ()  [unwired: 2 in, 2 out]
                n179 = property on="Ring" class="Ring (strict)"("Visible"=TRUE) -> ()  [unwired: 2 in, 2 out]
                n180 = property on="Slider" class="Slide (strict)"("Visible"=FALSE) -> ()  [unwired: 2 in, 2 out]
              }
              frame "Exposure Priority  **" {
                n181 = Index Array(array=w316, index=3) -> (element=w317:cluster{string[]})
                n182 = call <vilib>:"NT Read String.vi"("Name"=w319) -> ("String"=w318:string)  [unwired: 9 in, 1 out]
                n183 = Unbundle(w317) -> (w313:string[])
                n184 = Match First String(2:w313, 3:w318) -> (0:w314:i32)  [unwired: 1 out]
                n185 = property on="Ring" class="Ring (strict)"("Value"=w314, "Strings []"=w313) -> ()  [unwired: 2 in, 2 out]
                n186 = property on="Ring" class="Ring (strict)"("Visible"=TRUE) -> ()  [unwired: 2 in, 2 out]
                n187 = property on="Slider" class="Slide (strict)"("Visible"=FALSE) -> ()  [unwired: 2 in, 2 out]
              }
              frame "Color Enable  **" {
                n188 = Index Array(array=w325, index=4) -> (element=w326:cluster{string[]})
                n189 = call <vilib>:"NT Read String.vi"("Name"=w328) -> ("String"=w327:string)  [unwired: 9 in, 1 out]
                n190 = Unbundle(w326) -> (w322:string[])
                n191 = Match First String(2:w322, 3:w327) -> (0:w323:i32)  [unwired: 1 out]
                n192 = property on="Ring" class="Ring (strict)"("Value"=w323, "Strings []"=w322) -> ()  [unwired: 2 in, 2 out]
                n193 = property on="Ring" class="Ring (strict)"("Visible"=TRUE) -> ()  [unwired: 2 in, 2 out]
                n194 = property on="Slider" class="Slide (strict)"("Visible"=FALSE) -> ()  [unwired: 2 in, 2 out]
              }
              frame Default {
                n195 = property on="Ring" class="Ring (strict)"("Visible"=FALSE) -> ()  [unwired: 2 in, 2 out]
                n196 = property on="Slider" class="Slide (strict)"("Visible"=FALSE) -> ()  [unwired: 2 in, 2 out]
              }
              frame "Brightness  **", "Color Level  **", "Compression  **", "FPS  **", "Sharpness  **" {
                n197 = call <vilib>:"NT Read Number.vi"("Name"=w334) -> ("Numeric"=w333:dbl)  [unwired: 9 in, 1 out]
                n198 = local write "Slider"(w333) -> ()
                n199 = property on="Slider" class="Slide (strict)"("Visible"=TRUE, "Scale.Maximum"=100.0 ("Scale.Range:Maximum")) -> ()  [unwired: 2 in, 2 out]
                n200 = property on="Ring" class="Ring (strict)"("Visible"=FALSE) -> ()  [unwired: 2 in, 2 out]
              }
            }
          }
        }
        n201 = property on="Progress" class="Clust (strict)"("Visible"=FALSE) -> ()  [unwired: 2 in, 2 out]
      }
      event "Test Name": Mouse Enter {
        # "Populate the ring with the list of tests"
        n202 = event-data() -> ()  [unwired: 1 in, 1 out]
        n203 = call <vilib>:"NT Read String Array.vi"("Name"="TestMode/TestList") -> ("String Array"=w341:string[])  [unwired: 9 in, 1 out]
        n204 = Build Array (concatenate)("Select the test to run...", w341) -> (w340:string[])
        n205 = property on="Test Name" class="Ring (strict)"("Strings []"=w340) -> ()  [unwired: 2 in, 2 out]
      }
      event "Test Name": Value Change {
        w343 = FALSE ("Visible")
        # "Tell the robot the test name to run"
        n206 = event-data() -> ("NewVal"=w347:u16)  [unwired: 1 in]
        n207 = property on="Test Name" class="Ring (strict)"() -> ("Strings []"=w348:string[])  [unwired: 2 in, 2 out]
        n208 = local write "Progress"(T6 {"Test Progress"=0, "Test Progress Text"=""} ("Progress")) -> ()
        n209 = Index Array(array=w348, index=w347) -> (element=w346:string)
        n210 = call <vilib>:"NT Write String.vi"("String"=w346, "Name"="TestMode/TestName") -> ()  [unwired: 9 in, 1 out]
        n211 = property on="Progress" class="Clust (strict)"("Visible"=TRUE) -> ()  [unwired: 2 in, 2 out]
        n212 = property on="Motor" class="Clust (strict)"("Visible"=w343) -> ()  [unwired: 2 in, 2 out]
        n213 = property on="Slider" class="Slide (strict)"("Visible"=w343) -> ()  [unwired: 2 in, 2 out]
        n214 = property on="On/Off" class="Bool (strict)"("Visible"=w343) -> ()  [unwired: 2 in, 2 out]
        n215 = property on="Rev/Fwd" class="Clust (strict)"("Visible"=w343) -> ()  [unwired: 2 in, 2 out]
        n216 = property on="Ring" class="Ring (strict)"("Visible"=w343) -> ()  [unwired: 2 in, 2 out]
      }
      event "Listbox": Double Click {
        n217 = event-data() -> ("PlatMods.Shift"=w351:bool, "Row"=w353:i32)  [unwired: 1 in]
        n218 = case shown="False" w351 {
          tunnel: w353 -> [w357 _]
          tunnel: 1 -> [w356 _]
          frame False {
            n219 = property on="Listbox" class="LstBox (strict)"() -> ("Item Symbols"=w355:i32[])  [unwired: 2 in, 2 out]
            n220 = Replace Array Subset(array=w355, new element=w356, index=w357) -> (w354:i32[])
            n221 = property on="Listbox" class="LstBox (strict)"("Item Symbols"=w354) -> ()  [unwired: 2 in, 2 out]
          }
          frame True {
            w358 = 0 ("Top Row")
            n222 = property on="Listbox" class="LstBox (strict)"() -> ("Number of Rows"=w360:u32)  [unwired: 2 in, 2 out]
            n223 = Initialize Array(0, w360) -> (w359:i32[])
            n224 = property on="Listbox" class="LstBox (strict)"("Top Row"=w358, "Value"=w358, "Item Symbols"=w359) -> ()  [unwired: 2 in, 2 out]
          }
        }
      }
      event "Listbox": Key Down {
        n225 = event-data() -> ("VKey"=w364:T11)  [unwired: 1 in]
        n226 = case shown="\"Left\", \"Right\"" w364 {
          selector: w364 -> [w369 _]
          tunnel: eventvkey."Left" ("VKey") -> [w367 _]
          frame "Left", "Right" {
            n227 = Equal?(x=w367, y=w369) -> (x = y?=w368:bool)
            n228 = Select(t=0, s=w368, f=1) -> (s? t:f=w370:i32)
            n229 = property on="Listbox" class="LstBox (strict)"() -> ("Item Symbols"=w373:i32[])  [unwired: 2 in, 2 out]
            n230 = Replace Array Subset(array=w373, new element=w370, index="Listbox") -> (w372:i32[])
            n231 = property on="Listbox" class="LstBox (strict)"("Item Symbols"=w372) -> ()  [unwired: 2 in, 2 out]
          }
          frame Default {
          }
        }
      }
      event "DB Camera Config": Value Change {
        n232 = event-data() -> ("NewVal"=w377:bool)  [unwired: 1 in]
        n233 = case shown="False" w377 {
          tunnel: w376 -> [w386 _]
          tunnel: [w379 w397] -> w375
          tunnel: w374 -> [w378 w397]
          frame False {
            w393 = "Camera"
            w396 = FALSE ("Visible")
            n234 = local read "Camera Settings"() -> (w385:T3)
            n235 = Index Array(array=w386) -> (element=w389:cluster{string[]})  [unwired: 1 in]
            n236 = Unbundle(w385) -> ("Frame Rate"=w384:i32, "Compression"=w383:i32, "Size"=w387:u16)
            n237 = Unbundle(w389) -> (w388:string[])
            n238 = Index Array(array=w388, index=w387) -> (element=w382:string)
            n239 = call-poly <vilib>:"Write Key.vi"("section"=w393, "value"=w382, "key"="Size", "refnum"=w378) -> ("refnum out"=w395:T10)  [unwired: 2 in, 5 out]
            n240 = call-poly <vilib>:"Write Key.vi"("section"=w393, "value"=w384, "key"="FrameRate", "refnum"=w395) -> ("refnum out"=w394:T10)  [unwired: 1 in, 6 out]
            n241 = property on="Camera Settings" class="Clust (strict)"("Visible"=w396) -> ()  [unwired: 2 in, 2 out]
            n242 = local write "DB Camera Config"(w396) -> ()
            n243 = call-poly <vilib>:"Write Key.vi"("section"=w393, "value"=w383, "key"="Compression", "refnum"=w394) -> ("refnum out"=w380:T10)  [unwired: 1 in, 6 out]
            n244 = call <vilib>:"Close Config Data.vi"("refnum"=w380) -> ("file path"=w381:path)  [unwired: 2 in, 8 out]
            n245 = call <vilib>:"Open Config Data.vi"("configuration file path"=w381) -> ("refnum"=w379:T10)  [unwired: 8 in, 2 out]
          }
          frame True {
            n246 = property on="Camera Settings" class="Clust (strict)"("Visible"=TRUE) -> ()  [unwired: 2 in, 2 out]
          }
        }
      }
      event "Camera Settings": Value Change {
        n247 = event-data() -> ("NewVal"=w410:T3)  [unwired: 1 in]
        n248 = Index Array(array=w406) -> (element=w405:cluster{string[]})  [unwired: 1 in]
        n249 = Unbundle(w410) -> ("Frame Rate"=w401:i32, "Compression"=w400:i32, "Size"=w403:u16)
        n250 = Unbundle(w405) -> (w404:string[])
        n251 = Index Array(array=w404, index=w403) -> (element=w402:string)
        n252 = Format Into String(format string="%s   %dfps   %d%%", w402, w401, w400) -> (resulting string=w407:string)  [unwired: 2 in, 1 out]
        n253 = Build Array(w407) -> (w408:string[])
        n254 = property on="DB Camera Config" class="Bool (strict)"("Strings [4]"=w408) -> ()  [unwired: 2 in, 2 out]
      }
      event "Motor.Enable": Value Change {
        n255 = event-data() -> ("NewVal"=w416:bool)  [unwired: 1 in]
        n256 = Unbundle("Motor") -> ("Value"=w415:dbl)  [unwired: 1 out]
        n257 = Select(t=w415, s=w416, f=0.0) -> (s? t:f=w413:dbl)
        n258 = call <vilib>:"NT Write Number.vi"("Numeric"=w413, "Name"=w412) -> ()  [unwired: 9 in, 1 out]
      }
      event "Slider": Value Change {
        n259 = event-data() -> ("NewVal"=w419:dbl)  [unwired: 1 in]
        n260 = call <vilib>:"NT Write Number.vi"("Numeric"=w419, "Name"=w420) -> ()  [unwired: 9 in, 1 out]
      }
      event "On/Off": Value Change {
        n261 = event-data() -> ("NewVal"=w424:bool)  [unwired: 1 in]
        n262 = Boolean To (0,1)(Boolean=w424) -> (0, 1=w423:i16)
        n263 = call <vilib>:"NT Write Number.vi"("Numeric"=w423, "Name"=w422) -> ()  [unwired: 9 in, 1 out]
      }
      event "Rev/Fwd": Value Change {
        n264 = event-data() -> ("NewVal.Forward"=w432:bool, "NewVal.Reverse"=w431:bool)  [unwired: 1 in]
        n265 = Boolean To (0,1)(Boolean=w432) -> (0, 1=w428:i16)
        n266 = Boolean To (0,1)(Boolean=w431) -> (0, 1=w430:i16)
        n267 = Negate(x=w430) -> (-x=w429:i16)
        n268 = Add(x=w428, y=w429) -> (x+y=w427:i16)
        n269 = call <vilib>:"NT Write Number.vi"("Numeric"=w427, "Name"=w426) -> ()  [unwired: 9 in, 1 out]
      }
      event "Ring": Value Change {
        n270 = event-data() -> ("NewVal"=w436:u16)  [unwired: 1 in]
        n271 = property on="Ring" class="Ring (strict)"() -> ("Strings []"=w437:string[])  [unwired: 2 in, 2 out]
        n272 = Index Array(array=w437, index=w436) -> (element=w435:string)
        n273 = call <vilib>:"NT Write String.vi"("String"=w435, "Name"=w434) -> ()  [unwired: 9 in, 1 out]
      }
    }
  }
  n274 = Index Array(array=w17) -> (element=w18:cluster{string[]})  [unwired: 1 in]
  n275 = Unbundle(w18) -> (w16:string[])
  n276 = Match First String(2:w16, 3:w15) -> (0:w14:i32)  [unwired: 1 out]
  n277 = Bundle("value"=w20, "value"=w19, "index"=w14) -> (w8:cluster{"value":i32, "value":i32, "index":i32})  [unwired: 1 out]
  n278 = property on="On/Off" class="Bool (strict)"("Visible"=w31) -> ()  [unwired: 2 in, 2 out]
  n279 = property on="Motor" class="Clust (strict)"("Visible"=w31) -> ()  [unwired: 2 in, 2 out]
  n280 = property on="Camera Settings" class="Clust (strict)"("Val(Sgnl)"=w8) -> ()  [unwired: 2 in, 2 out]
  n281 = property on="Rev/Fwd" class="Clust (strict)"("Visible"=w31) -> ()  [unwired: 2 in, 2 out]
  n282 = property on="Progress" class="Clust (strict)"("Visible"=w31) -> ()  [unwired: 2 in, 2 out]
  n283 = property on="Camera Settings" class="Clust (strict)"("Visible"=w31) -> ()  [unwired: 2 in, 2 out]
  n284 = local write "DB Camera Config"(w31) -> ()
  n285 = property on="Ring" class="Ring (strict)"("Visible"=w31) -> ()  [unwired: 2 in, 2 out]
